vi "Get Inputs Definition.vi"(11 "Inputs":refnum<class "Terminal.lvclass">[](array[class])) -> (2 "Default Input":variant, 3 "input string":string)   [LabVIEW 2019, in "Terminal.lvclass"]
doc: "JKI State Machine Objects (SMO) 1.3.0.56\nJKI - JKI\nCopyright (c) 2017, JKI"
uses:
  Terminal.lvclass
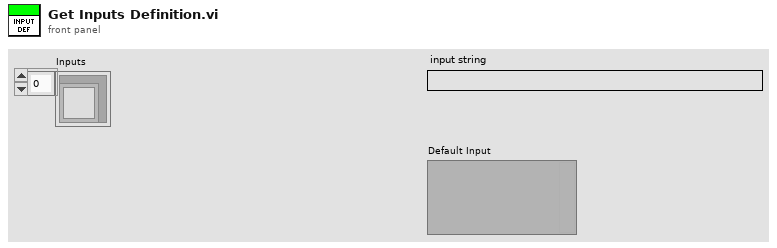
[diagram p1: front panel]
types:
  T1 = typedef "VariantType.lvlib/Type.ctl" = enum8{"Invalid Type", "Void", "I8", "I16", "I32", "I64", "U8", "U16", "U32", "U64", "Single Float", "Double Float", "Extended Float", "Single Complex", "Double Complex", "Extended Complex", "Enum U8", "Enum U16", "Enum U32", "Enum U64", "Single Float With Unit", "Double Float With Unit", "Extended Float With Unit", "Single Complex with Unit", "Double Complex with Unit", "Extended Complex with Unit", "Boolean", "String", "Path", "Picture", "Tag", "Array", "Cluster", "Variant", "LV Variant", "Waveform", "Timestamp", "Digital Waveform", "Digital Data", "ExpressData", "Refnum", "External Data", "VI", "Poly VI", "LabVIEW Class Instance", "Fixed Point"}
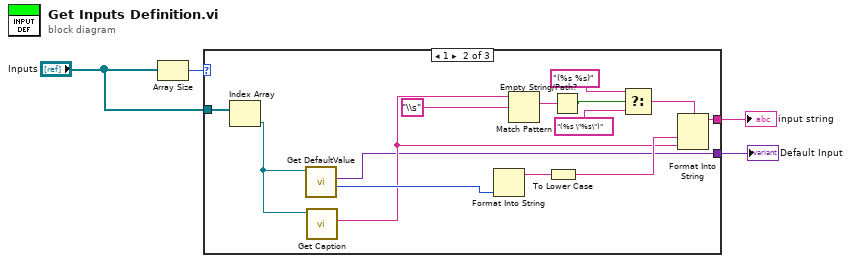
[diagram p0: block diagram]
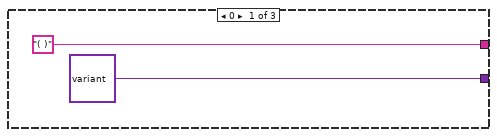
[diagram p2: hidden frame]
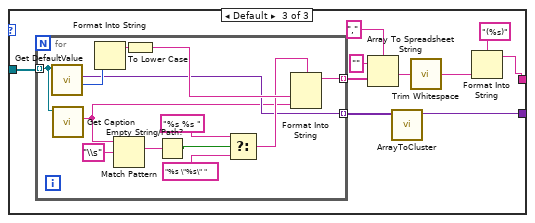
[diagram p3: hidden frame]
diagram:
  n1 = Array Size(array="Inputs") -> (size(s)=w4:i32)
  n2 = case shown="1" w4 {
    tunnel: "Inputs" -> [_ w20 w30]
    tunnel: ["( )" w19 w27] -> w2
    tunnel: [variant ("Default Value") w7 w21] -> w1
    frame 0 {
    }
    frame 1 {
      n3 = Index Array(array=w20) -> (element=w10:refnum<class "Terminal.lvclass">)  [unwired: 1 in]
      n4 = call "Get DefaultValue.vi"("Terminal in"=w10) -> ("Type Enum"=w9:T1, "Default Value"=w7:variant)  [unwired: 7 in, 2 out]
      n5 = call "Get Caption.vi"("Terminal in"=w10) -> ("Caption"=w8:string)  [unwired: 8 in, 2 out]
      n6 = Format Into String(w9) -> (resulting string=w18:string)  [unwired: 3 in, 1 out]
      n7 = Match Pattern(string=w8, regular expression="\\s") -> (match substring=w15:string)  [unwired: 1 in, 3 out]
      n8 = To Lower Case(string=w18) -> (all lower case string=w17:string)
      n9 = Empty String/Path?(string/path=w15) -> (empty?=w14:bool)
      n10 = Select(t="(%s %s)" ("format string"), s=w14, f="(%s \"%s\")" ("format string")) -> (s? t:f=w12:string)
      n11 = Format Into String(format string=w12, w17, w8) -> (resulting string=w19:string)  [unwired: 2 in, 1 out]
    }
    frame Default {
      n12 = for {
        tunnel: [w43] -> w29 mode=indexing
        tunnel: w30 -> [w32] mode=indexing
        tunnel: [w33] -> w22 mode=indexing
        n13 = call "Get DefaultValue.vi"("Terminal in"=w32) -> ("Type Enum"=w34:T1, "Default Value"=w33:variant)  [unwired: 7 in, 2 out]
        n14 = call "Get Caption.vi"("Terminal in"=w32) -> ("Caption"=w31:string)  [unwired: 8 in, 2 out]
        n15 = Format Into String(w34) -> (resulting string=w42:string)  [unwired: 3 in, 1 out]
        n16 = Match Pattern(string=w31, regular expression="\\s") -> (match substring=w39:string)  [unwired: 1 in, 3 out]
        n17 = To Lower Case(string=w42) -> (all lower case string=w41:string)
        n18 = Empty String/Path?(string/path=w39) -> (empty?=w38:bool)
        n19 = Select(t="%s %s " ("format string"), s=w38, f="%s \"%s\" " ("format string")) -> (s? t:f=w35:string)
        n20 = Format Into String(format string=w35, w41, w31) -> (resulting string=w43:string)  [unwired: 2 in, 1 out]
      }
      n21 = Array To Spreadsheet String(delimiter (Tab)=",", array=w29, 3:"" ("format string")) -> (spreadsheet string=w28:string)
      n22 = call "ArrayToCluster.vi"("Array"=w22) -> ("Cluster"=w21:variant)  [unwired: 10 in]
      n23 = call <vilib>:"Trim Whitespace.vi"("string"=w28) -> ("trimmed string"=w23:string)  [unwired: 1 in]
      n24 = Format Into String(format string="(%s)", w23) -> (resulting string=w27:string)  [unwired: 2 in, 1 out]
    }
  }
  "Default Input" <- w1
  "input string" <- w2
